vi "Execute.InitializeSequence.vi"(8 "error in (no error)":errorcluster, 11 "State Variables":T1={"NIVS.BaseLogPath"=path "", "NIVS.SystemDefinitionFile"=path "", "NIVS.Events"={"SequenceEvent"=refnum, "SystemChangeEvent"=refnum, "WorkspaceEvent"=refnum}, "NIVS.SequenceState"=enum."Idle", "NIVS.GatewayIPAddress"="", "NIVS.DataLogSpecRef"=refnum, "NIVS.DataLogManagerRef"=refnum, "NIVS.LogSessionGUID"="", "NIVS.WorkspaceManager"=refnum, "NIVS.Deployed"=FALSE, "NIVS.ProfileRef"=refnum, "NIVS.ProfileCallback"=refnum, "NIVS.SystemStateRefs"={"CustDatRef"=refnum, "EvtRef"=refnum}, "UI.Abort"=refnum, "UI.Pause"=refnum, "UI.EnableLogging"=refnum, "UI.Start"=refnum, "UI.LogChannels"=refnum, "UI.StartIteration"=refnum, "UI.StartStep"=refnum, "UI.Sequence"=refnum, "UI.PreviewMode"=refnum, "UI.Graph"=refnum, "UI.BaseFileName"=refnum, "UI.Profiles"=refnum, "UI.CurrentStep"=refnum, "UI.CurrentIteration"=refnum, "UI.TotalIterations"=refnum, "Sequence.AbortChannel"="", "Sequence.StepInfoChannel"="", "Sequence.Iterations"=0, "Sequence.IterationInfoChannel"="", "Sequence.#ofColumns"=0, "Events.State"=refnum, "Events.Test Result"=refnum, "Events.Progress"=refnum, "INI.Settings"={"Build Location"=path "C:/Simple Sequence Editor/SequenceRepo", "LoggingLocation"=path ""}}) -> (0 "error out":errorcluster, 3 "State Variables":T1={"NIVS.BaseLogPath"=path "", "NIVS.SystemDefinitionFile"=path "", "NIVS.Events"={"SequenceEvent"=refnum, "SystemChangeEvent"=refnum, "WorkspaceEvent"=refnum}, "NIVS.SequenceState"=enum."Idle", "NIVS.GatewayIPAddress"="", "NIVS.DataLogSpecRef"=refnum, "NIVS.DataLogManagerRef"=refnum, "NIVS.LogSessionGUID"="", "NIVS.WorkspaceManager"=refnum, "NIVS.Deployed"=FALSE, "NIVS.ProfileRef"=refnum, "NIVS.ProfileCallback"=refnum, "NIVS.SystemStateRefs"={"CustDatRef"=refnum, "EvtRef"=refnum}, "UI.Abort"=refnum, "UI.Pause"=refnum, "UI.EnableLogging"=refnum, "UI.Start"=refnum, "UI.LogChannels"=refnum, "UI.StartIteration"=refnum, "UI.StartStep"=refnum, "UI.Sequence"=refnum, "UI.PreviewMode"=refnum, "UI.Graph"=refnum, "UI.BaseFileName"=refnum, "UI.Profiles"=refnum, "UI.CurrentStep"=refnum, "UI.CurrentIteration"=refnum, "UI.TotalIterations"=refnum, "Sequence.AbortChannel"="", "Sequence.StepInfoChannel"="", "Sequence.Iterations"=0, "Sequence.IterationInfoChannel"="", "Sequence.#ofColumns"=0, "Events.State"=refnum, "Events.Test Result"=refnum, "Events.Progress"=refnum, "INI.Settings"={"Build Location"=path "C:/Simple Sequence Editor/SequenceRepo", "LoggingLocation"=path ""}})   [LabVIEW 2013, in "Simple Sequence Tools - Execution.lvlib"]
uses:
  Simple Sequence Tools - Execution.lvlib
  Types/Main.StateVariables.ctl
  Types/Execute.UserEventRefs.ctl
  <vilib>/NI Veristand/Execution/Workspace/SystemStateRegEventRef.ctl
  Types/Execution.SequenceState.ctl
  <vilib>/NI Veristand/Execution/DataLogging/DataLoggingSpecification Ref.ctl
  NationalInstruments.VeriStand.ClientAPI
  <vilib>/NI Veristand/Execution/DataLogging/IDataLogging Ref.ctl
  <vilib>/NI Veristand/Execution/Workspace/WorkspaceAPI.ctl
  NationalInstruments.VeriStand.RealTimeSequenceDefinitionApi
  <vilib>/NI Veristand/Execution/Workspace/SystemStateEventRef.ctl
  Shared/Types/INI.Settings
  Shared/SubVIs/Main.Constants.vi
  Shared/Simple Sequence Tools - Shared.lvlib
  <vilib>/NI Veristand/Execution/Workspace/NI_VS Workspace ExecutionAPI.lvlib
  <vilib>/NI Veristand/Execution/DataLogging/NI_VS Data Logging API.lvlib
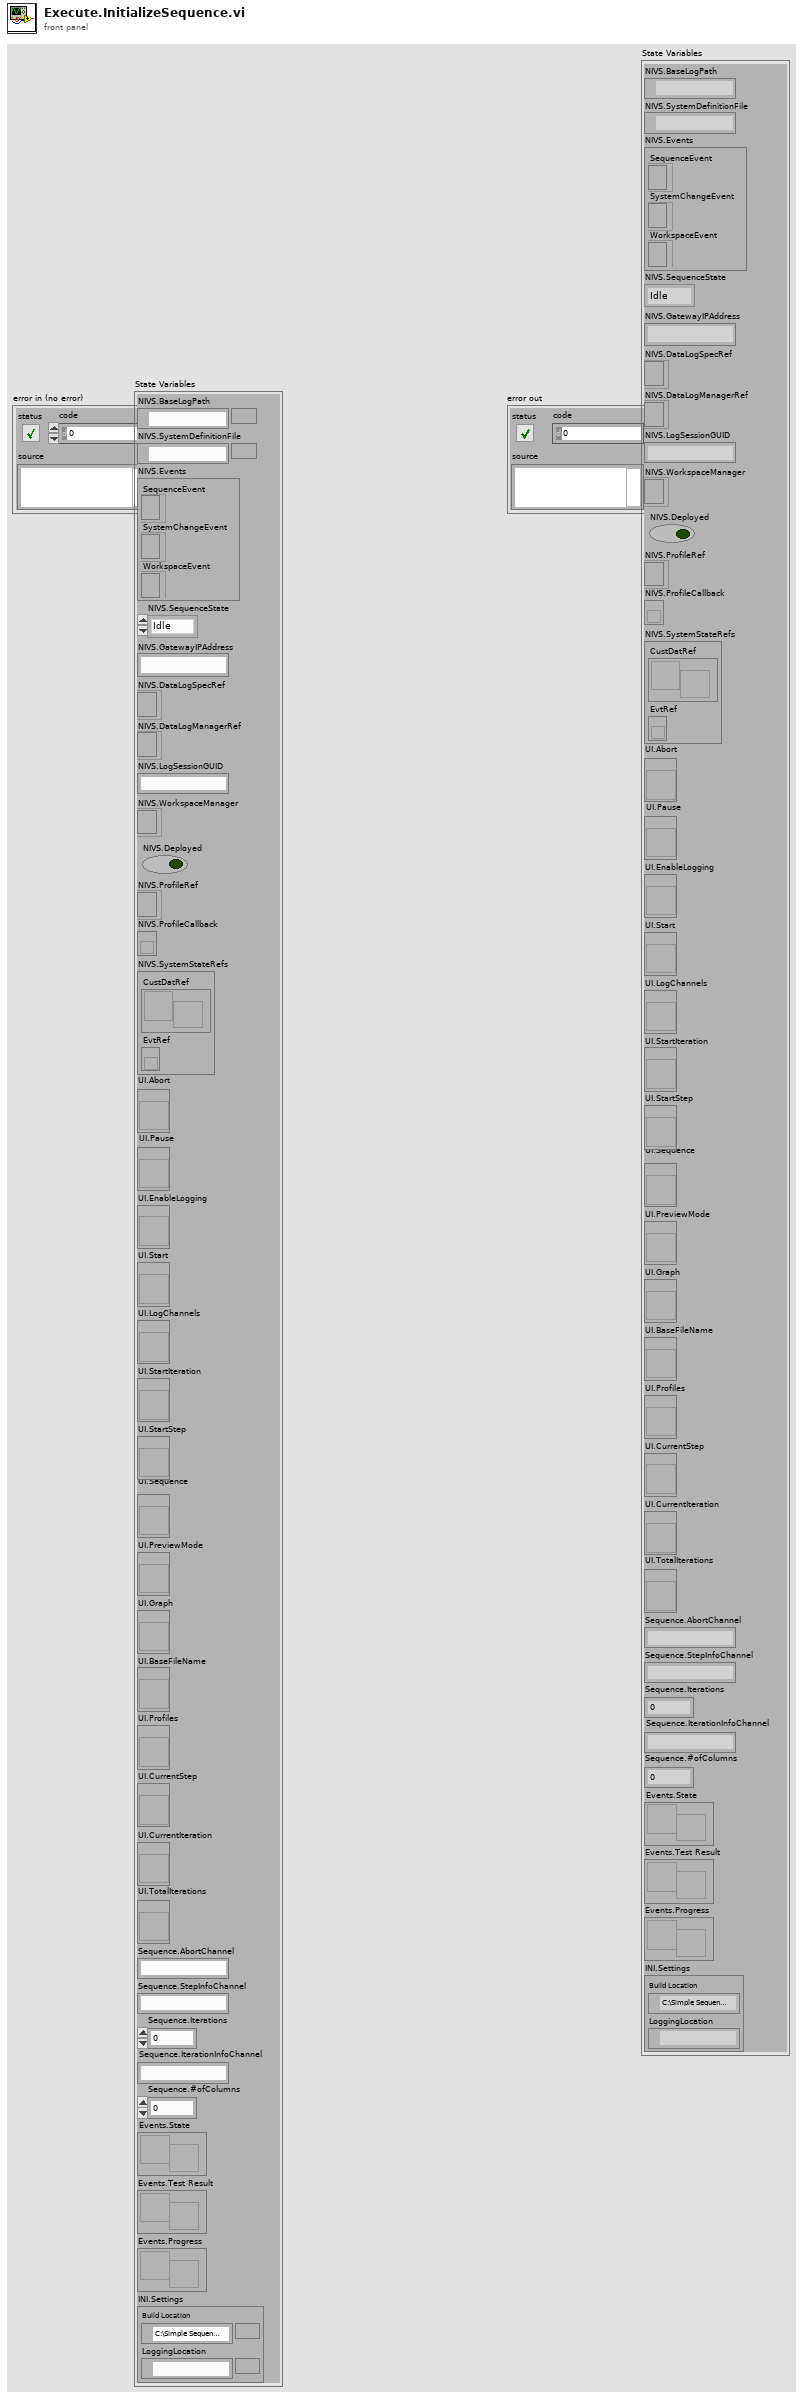
[diagram p1: front panel]
types:
  T1 = typedef "Simple Sequence Tools - Execution.lvlib/Main.StateVariables.ctl" = cluster{"NIVS.BaseLogPath":path, "NIVS.SystemDefinitionFile":path, "NIVS.Events":T2, "NIVS.SequenceState":T4, "NIVS.GatewayIPAddress":string, "NIVS.DataLogSpecRef":T5, "NIVS.DataLogManagerRef":T6, "NIVS.LogSessionGUID":string, "NIVS.WorkspaceManager":T7, "NIVS.Deployed":bool, "NIVS.ProfileRef":refnum<k24>, "NIVS.ProfileCallback":refnum<k27>, "NIVS.SystemStateRefs":T8, "UI.Abort":refnum<vi>, "UI.Pause":refnum<vi>, "UI.EnableLogging":refnum<vi>, "UI.Start":refnum<vi>, "UI.LogChannels":refnum<vi>, "UI.StartIteration":refnum<vi>, "UI.StartStep":refnum<vi>, "UI.Sequence":refnum<vi>, "UI.PreviewMode":refnum<vi>, "UI.Graph":refnum<vi>, "UI.BaseFileName":refnum<vi>, "UI.Profiles":refnum<vi>, "UI.CurrentStep":refnum<vi>, "UI.CurrentIteration":refnum<vi>, "UI.TotalIterations":refnum<vi>, "Sequence.AbortChannel":string, "Sequence.StepInfoChannel":string, "Sequence.Iterations":u32, "Sequence.IterationInfoChannel":string, "Sequence.#ofColumns":i32, "Events.State":refnum<user-event>, "Events.Test Result":refnum<user-event>, "Events.Progress":refnum<user-event>, "INI.Settings":T9}
  T2 = typedef "Simple Sequence Tools - Execution.lvlib/Execute.UserEventRefs.ctl" = cluster{"SequenceEvent":refnum<event-registration>, "SystemChangeEvent":T3, "WorkspaceEvent":refnum<event-registration>}
  T3 = typedef "NI_VS Workspace ExecutionAPI.lvlib/SystemStateRegEventRef.ctl" = refnum<event-registration>
  T4 = typedef "Simple Sequence Tools - Execution.lvlib/Execution.SequenceState.ctl" = enum16{"Idle", "Initializing", "Running", "Paused", "Finalizing", "Complete"}
  T5 = typedef "NI_VS Data Logging API.lvlib/DataLoggingSpecification Ref.ctl" = refnum<k24>
  T6 = typedef "NI_VS Data Logging API.lvlib/IDataLogging Ref.ctl" = refnum<k24>
  T7 = typedef "NI_VS Workspace ExecutionAPI.lvlib/WorkspaceAPI.ctl" = refnum<k24>
  T8 = typedef "NI_VS Workspace ExecutionAPI.lvlib/SystemStateEventRef.ctl" = cluster{"CustDatRef":refnum<user-event>, "EvtRef":refnum<k27>}
  T9 = typedef "Simple Sequence Tools - Shared.lvlib/INI.Settings" = cluster{"Build Location":path, "LoggingLocation":path}
  T10 = enum8{"Enabled", "Disabled", "Disabled and Grayed Out"}
  T11 = typedef "Simple Sequence Tools - Shared.lvlib/Saved.Sequence.ctl" = cluster{"Output Channels":T12[], "Item Names":string[][], "Step":string, "Abort":string, "Iterations":u32, "Iteration":string}
  T12 = typedef "Simple Sequence Tools - Shared.lvlib/Channel.Properties.ctl" = cluster{"Name":string, "NodePath":string, "ScaleUnits":string}
  T13 = typedef "LVBoundsTypeDef.ctl" = cluster{"Width":u32, "Height":u32}
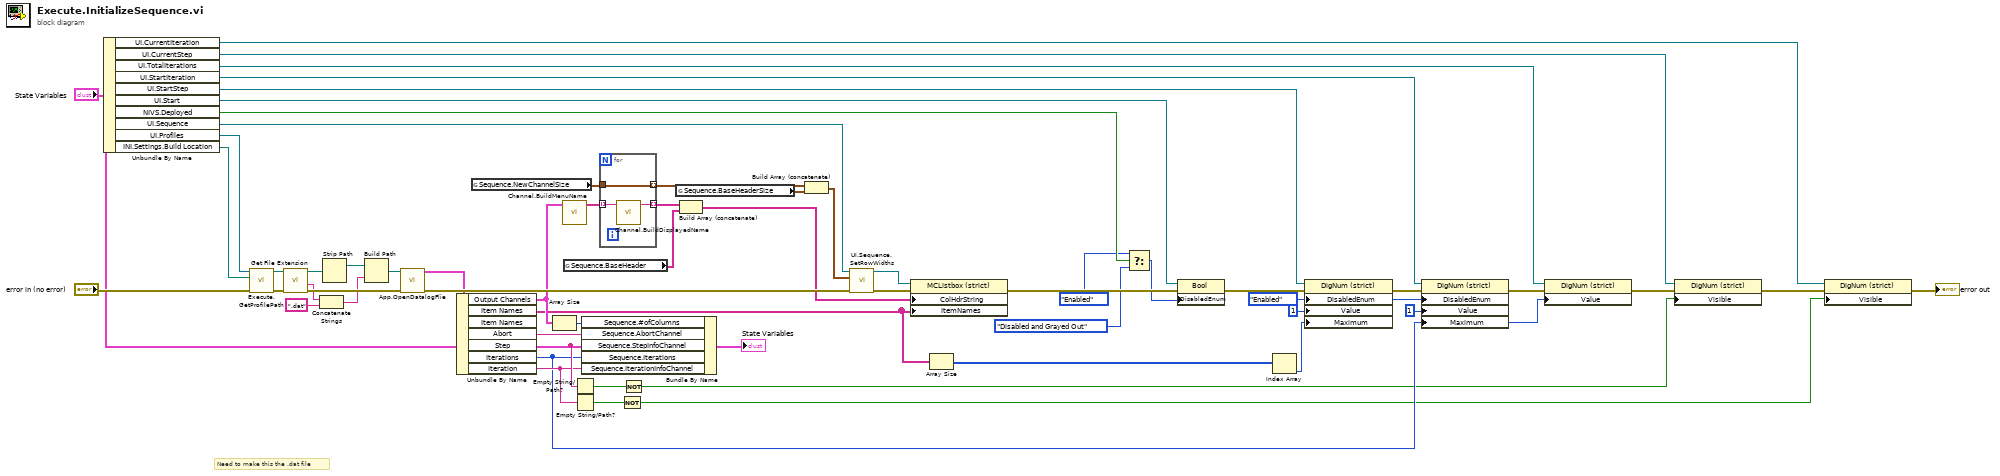
[diagram p0: block diagram]
diagram:
  w24 = T10."Enabled" ("Disabled")
  # "Need to make this the .dat file"
  n1 = Unbundle By Name("State Variables") -> ("UI.CurrentIteration"=w15:refnum<vi>, "UI.CurrentStep"=w16:refnum<vi>, "UI.TotalIterations"=w4:refnum<vi>, "UI.StartIteration"=w25:refnum<vi>, "UI.StartStep"=w9:refnum<vi>, "UI.Start"=w41:refnum<vi>, "NIVS.Deployed"=w39:bool, "UI.Sequence"=w49:refnum<vi>, "UI.Profiles"=w26:refnum<vi>, "INI.Settings.Build Location"=w1:path)
  n2 = call "Execute.GetProfilePath.vi"("error in (no error)"="error in (no error)", "base path"=w1, "Profiles"=w26) -> ("error out"=w33:errorcluster, "Path"=w35:path)  [unwired: 7 in]
  n3 = call <vilib>:"Get File Extension.vi"("error in (no error)"=w33, "file"=w35) -> ("error out"=w32:errorcluster, "filename without extension"=w30:string, "dup file"=w34:path)  [unwired: 6 in, 1 out]
  n4 = Concatenate Strings(w30, ".dat" ("string")) -> (w28:string)
  n5 = Strip Path(path=w34) -> (stripped path=w31:path)  [unwired: 1 out]
  n6 = Build Path(base path=w31, name or relative path=w28) -> (appended path=w27:path)
  n7 = call "App.OpenDatalogFlie.vi"("error in (no error)"=w32, "selected path"=w27) -> ("error out"=w58:errorcluster, "Settings"=w47:T11)  [unwired: 8 in]
  n8 = Unbundle By Name(w47) -> ("Output Channels"=w42:T12[], "Item Names"=w22:string[][], "Abort"=w45:string, "Step"=w14:string, "Iterations"=w5:u32, "Iteration"=w13:string)  [unwired: 1 out]
  n9 = global read "Main.Constants.vi" "Sequence.NewChannelSize"() -> (w54:T13)
  n10 = Array Size(array=w42) -> (size(s)=w43:i32)
  n11 = call "Channel.BuildMenuName.vi"("Aliases"=w42) -> ("Aliases Array"=w50:string[])  [unwired: 10 in]
  n12 = global read "Main.Constants.vi" "Sequence.BaseHeader"() -> (w53:string[])
  n13 = Empty String/Path?(string/path=w14) -> (empty?=w11:bool)
  n14 = Empty String/Path?(string/path=w13) -> (empty?=w12:bool)
  n15 = Bundle By Name(cluster="State Variables", "Sequence.#ofColumns"=w43, "Sequence.AbortChannel"=w45, "Sequence.StepInfoChannel"=w14, "Sequence.Iterations"=w5, "Sequence.IterationInfoChannel"=w13) -> (→"State Variables":T1)
  n16 = for {
    tunnel: w50 -> [w63] mode=indexing
    tunnel: [w62] -> w52 mode=indexing
    tunnel: [w61] -> w55 mode=indexing
    tunnel: w54 -> [w61]
    n17 = call "Channel.BuildDisplayedName.vi"("Path"=w63) -> ("Formated Path"=w62:string)  [unwired: 10 in]
  }
  n18 = Not(x=w12) -> (.not. x?=w2:bool)
  n19 = Not(x=w11) -> (.not. x?=w3:bool)
  n20 = global read "Main.Constants.vi" "Sequence.BaseHeaderSize"() -> (w56:T13[])
  n21 = Build Array (concatenate)(w52, w53) -> (w51:string[])
  n22 = Build Array (concatenate)(w55, w56) -> (w57:T13[])
  n23 = call "UI.Sequence.SetRowWidths.vi"("error in (no error)"=w58, "CellSize"=w57, "UI.SequenceRef"=w49) -> ("error out"=w59:errorcluster, "UI.SequenceRef"=w60:refnum<vi>)  [unwired: 7 in]
  n24 = property class="MCListbox (strict)"(reference=w60, error in=w59, "ColHdrString"=w51, "ItemNames"=w22) -> (error out=w40:errorcluster)  [unwired: 1 out]
  n25 = Array Size(array=w22) -> (size(s)=w21:i32[])
  n26 = Select(t=T10."Enabled" ("Disabled"), s=w39, f=T10."Disabled and Grayed Out" ("Disabled")) -> (s? t:f=w36:T10)
  n27 = property class="Bool"(reference=w41, error in=w40, "DisabledEnum"=w36) -> (error out=w10:errorcluster)  [unwired: 1 out]
  n28 = Index Array(array=w21) -> (element=w20:i32)  [unwired: 1 in]
  n29 = property class="DigNum (strict)"(reference=w9, error in=w10, "DisabledEnum"=w24, "Value"=u32 1, "Maximum"=w20) -> (error out=w8:errorcluster)  [unwired: 1 out]
  n30 = property class="DigNum (strict)"(reference=w25, error in=w8, "DisabledEnum"=w24, "Value"=u32 1, "Maximum"=w5) -> (error out=w7:errorcluster)  [unwired: 1 out]
  n31 = property class="DigNum (strict)"(reference=w4, error in=w7, "Value"=w5) -> (error out=w6:errorcluster)  [unwired: 1 out]
  n32 = property class="DigNum (strict)"(reference=w16, error in=w6, "Visible"=w3) -> (error out=w18:errorcluster)  [unwired: 1 out]
  n33 = property class="DigNum (strict)"(reference=w15, error in=w18, "Visible"=w2) -> (error out=→"error out":errorcluster)  [unwired: 1 out]
